vi "Main Page.vi"(8 "error in (no error)":errorcluster, 11 "Node Ptr":T1 format="%.0x") -> (0 "error out":errorcluster)   [LabVIEW 2017, in "NI-SWITCH System Explorer.lvlib"]
uses:
  NI-SWITCH System Explorer.lvlib
  <vilib>/NI Veristand/Custom Device API/Custom Device Item Ref.ctl
  Main Page Controls.ctl
  <vilib>/NI VeriStand/Custom Device API/Custom Device API.lvlib
  Scripting/NI-SWITCH Scripting.lvlib
panel:
  out "Normally Connected Information":cluster{"String":string}={"String"="This topology contains endpoints which are normally connected. See the documentation for more information."}
  in  "Custom Device Name":string
  in  "Topology":string(combo)
  in  "Resource":string
  in  "SHDocVw.IWebBrowser":refnum<k7>(container)
  in  "Description":string
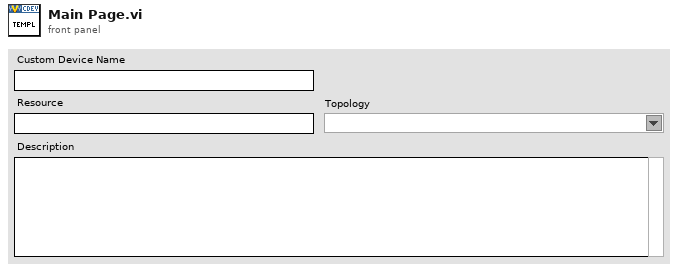
[diagram p1: front panel]
types:
  T1 = typedef "Custom Device API.lvlib/Custom Device Item Ref.ctl" = u64
  T2 = typedef "NI-SWITCH System Explorer.lvlib/Main Page Controls.ctl" = cluster{"Name":refnum<vi>, "Description":refnum<vi>, "Resource":refnum<vi>, "Topology":refnum<vi>, "Normally Connected Information":refnum<vi>}
  T3 = typedef "Custom Device API.lvlib/Custom Device Commands.ctl" = enum16{"Default", "Item renamed", "Shutdown", "Dynamic button pressed"}
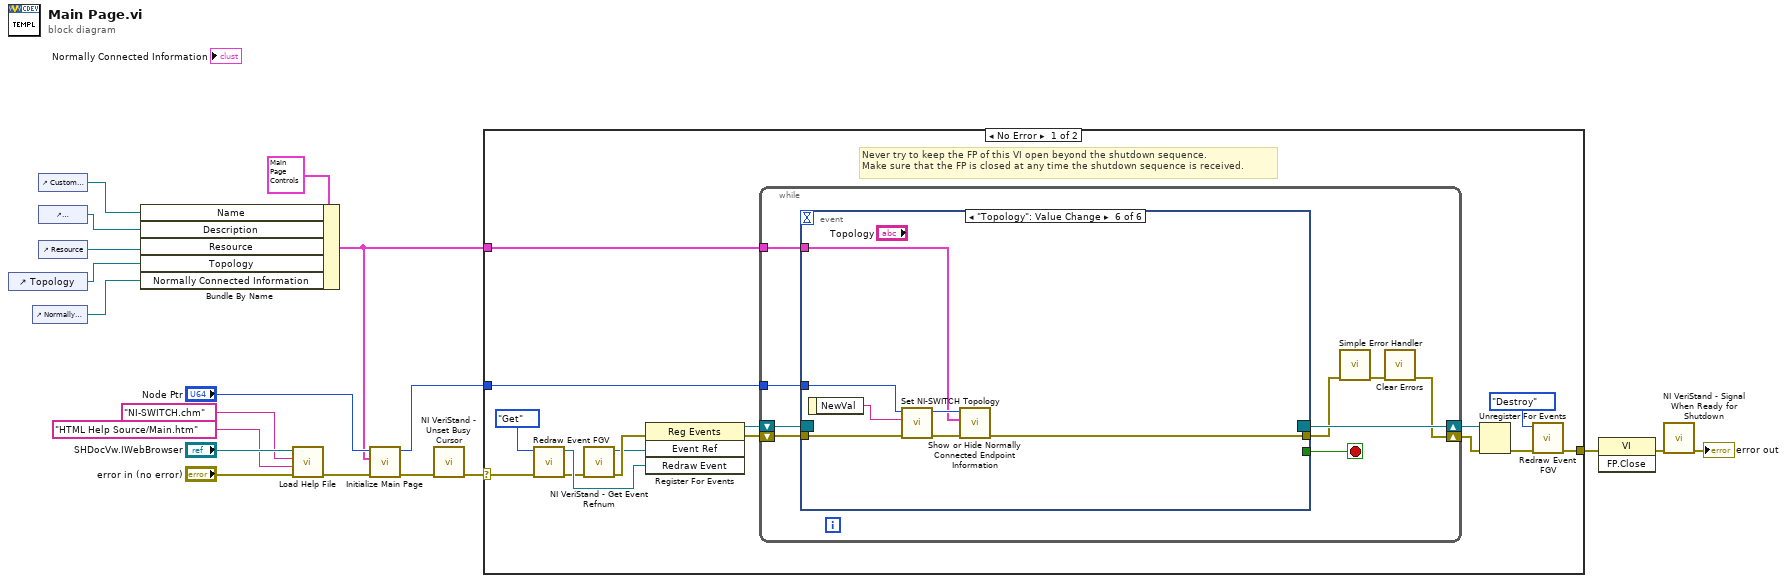
[diagram p0: block diagram]
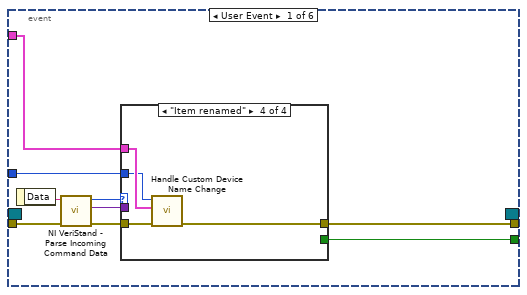
[diagram p2: hidden frame]
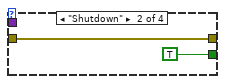
[diagram p4: hidden frame]
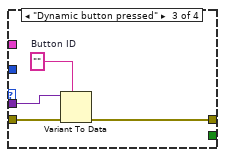
[diagram p5: hidden frame]
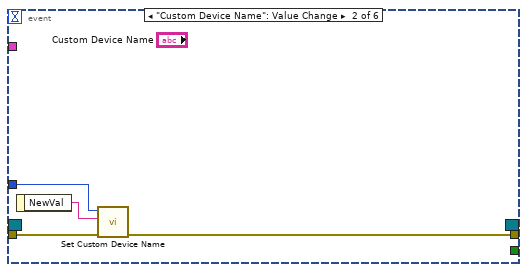
[diagram p6: hidden frame]
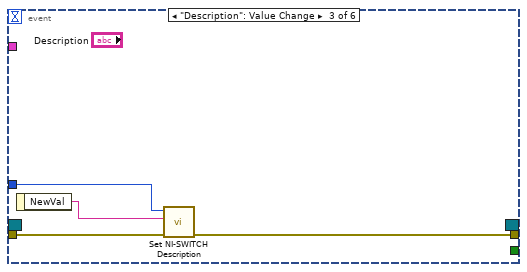
[diagram p7: hidden frame]
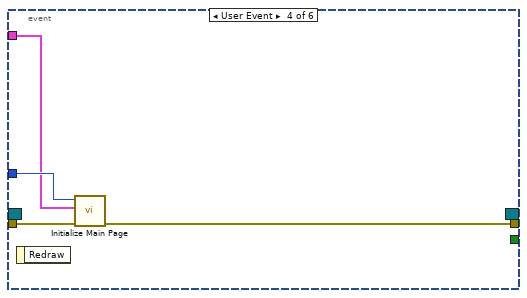
[diagram p8: hidden frame]
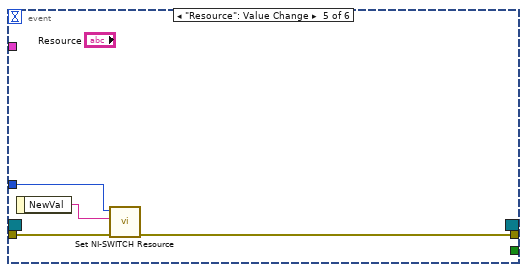
[diagram p9: hidden frame]
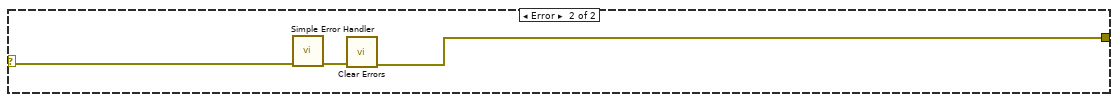
[diagram p10: hidden frame]
diagram:
  n1 = control-ref of="Topology"() -> (w5:refnum<vi>)
  n2 = control-ref of="Normally Connected Information"() -> (w1:refnum<vi>)
  n3 = control-ref of="Custom Device Name"() -> (w2:refnum<vi>)
  n4 = control-ref of="Description"() -> (w8:refnum<vi>)
  n5 = control-ref of="Resource"() -> (w4:refnum<vi>)
  n6 = Bundle By Name(cluster=T2 {"Name"=refnum, "Description"=refnum, "Resource"=refnum, "Topology"=refnum, "Normally Connected Information"=refnum} ("Main Page Controls"), "Name"=w2, "Description"=w8, "Resource"=w4, "Topology"=w5, "Normally Connected Information"=w1) -> (w3:T2)
  n7 = call "Load Help File.vi"("error in (no error)"="error in (no error)", "HTML File to Load"="HTML Help Source/Main.htm" ("HTML File"), "Main CHM File"="NI-SWITCH.chm" ("CD_CHM_FileName"), "Browser"="SHDocVw.IWebBrowser") -> ("error out"=w6:errorcluster)  [unwired: 7 in]
  n8 = call "Initialize Main Page.vi"("error in (no error)"=w6, "Main Page Controls"=w3, "Item Ref in"="Node Ptr") -> ("error out"=w15:errorcluster, "Item Ref out"=w12:T1)  [unwired: 7 in]
  n9 = call <vilib>:"NI VeriStand - Unset Busy Cursor.vi"("error in (no error)"=w15) -> ("error out"=w14:errorcluster)  [unwired: 10 out]
  n10 = case shown="No Error" w14 {
    selector: w14 -> [w22 w89]
    tunnel: [w24 w87] -> w19
    tunnel: w12 -> [w28 _]
    tunnel: w3 -> [w26 _]
    frame No Error {
      # "Never try to keep the FP of this VI open beyond the shutdown sequence.\nMake sure that the FP is closed at any time the shutdown sequence is received."
      n11 = call "Redraw Event FGV.vi"("error in (no error)"=w22, "Action (Get)"=enum16{"Get", "Destroy"}."Get") -> ("error out"=w21:errorcluster, "Redraw Event"=w27:refnum<user-event>)  [unwired: 8 in]
      n12 = call <vilib>:"NI VeriStand - Get Event Refnum.vi"("error in (no error)"=w21) -> ("error out"=w34:errorcluster, "Event Ref"=w31:refnum<user-event>)  [unwired: 9 out]
      n13 = register-events(error in=w34, w31, w27) -> (reference out=w29:refnum<event-registration>, error out=w30:errorcluster)  [unwired: 1 in]
      n14 = while {
        tunnel: w28 -> [w39]
        shift-right: [w36] -> w32
        shift-left: w30 -> [w42]
        shift-right: [w43] -> w33
        shift-left: w29 -> [w41]
        tunnel: w26 -> [w35]
        stop <- w40 stop-if-true
        n15 = event shown="[5] \"Topology\": Value Change" {
          selector: w41 -> [_ _ _ _ _ _]
          dyn-events: [_ _ _ _ _ _] -> w43
          timeout: _ -> [_ _ _ _ _ _]
          tunnel: w42 -> [w52 w67 w70 w73 w79 w86]
          tunnel: [w48 _ _ _ _ _] -> w40
          tunnel: [w47 w66 w69 w72 w76 w82] -> w38
          tunnel: w39 -> [w46 w65 w71 w75 w78 w85]
          tunnel: w35 -> [w44 _ _ w74 _ w80]
          event User Event {
            n16 = event-data() -> ("Data"=w51:string)  [unwired: 1 out]
            n17 = call <vilib>:"NI VeriStand - Parse Incoming Command Data.vi"("error in (no error)"=w52, "Incoming data"=w51) -> ("error out"=w50:errorcluster, "Outgoing data"=w45:variant, "Action"=w49:T3)  [unwired: 7 out]
            n18 = case shown="\"Item renamed\"" w49 {
              tunnel: w50 -> [w53 w54 w59 w63]
              tunnel: [_ TRUE _ _] -> w48
              tunnel: [w53 w54 w56 w62] -> w47
              tunnel: w46 -> [_ _ _ w60]
              tunnel: w45 -> [_ _ w58 _]
              tunnel: w44 -> [_ _ _ w61]
              frame "Default", Default {
              }
              frame "Shutdown" {
              }
              frame "Dynamic button pressed" {
                w57 = ""  # Button ID
                n19 = Variant To Data(error in=w59, type=w57, Variant=w58) -> (error out=w56:errorcluster)  [unwired: 1 out]
              }
              frame "Item renamed" {
                n20 = call "Handle Custom Device Name Change.vi"("error in (no error)"=w63, "Main Page Controls"=w61, "Item Ref in"=w60) -> ("error out"=w62:errorcluster)  [unwired: 7 in, 1 out]
              }
            }
          }
          event "Custom Device Name": Value Change {
            n21 = event-data() -> ("NewVal"=w64:string)  [unwired: 1 out]
            n22 = call "Set Custom Device Name.vi"("error in"=w67, "name"=w64, "ni-switch custom device in"=w65) -> ("error out"=w66:errorcluster)  [unwired: 6 in, 1 out]
          }
          event "Description": Value Change {
            n23 = event-data() -> ("NewVal"=w68:string)  [unwired: 1 out]
            n24 = call "Set NI-SWITCH Description.vi"("error in"=w70, "description"=w68, "ni-switch custom device in"=w71) -> ("error out"=w69:errorcluster)  [unwired: 7 in, 1 out]
          }
          event User Event {
            n25 = event-data() -> ()  [unwired: 2 out]
            n26 = call "Initialize Main Page.vi"("error in (no error)"=w73, "Main Page Controls"=w74, "Item Ref in"=w75) -> ("error out"=w72:errorcluster)  [unwired: 7 in, 1 out]
          }
          event "Resource": Value Change {
            n27 = event-data() -> ("NewVal"=w77:string)  [unwired: 1 out]
            n28 = call "Set NI-SWITCH Resource.vi"("error in"=w79, "resource"=w77, "ni-switch custom device in"=w78) -> ("error out"=w76:errorcluster)  [unwired: 7 in, 1 out]
          }
          event "Topology": Value Change {
            n29 = event-data() -> ("NewVal"=w84:string)  [unwired: 1 out]
            n30 = call "Set NI-SWITCH Topology.vi"("error in"=w86, "topology"=w84, "ni-switch custom device in"=w85) -> ("error out"=w83:errorcluster, "ni-switch custom device out"=w81:T1)  [unwired: 7 in]
            n31 = call "Show or Hide Normally Connected Endpoint Information.vi"("error in (no error)"=w83, "Main Page Controls"=w80, "ni-switch custom device in"=w81) -> ("error out"=w82:errorcluster)  [unwired: 7 in, 1 out]
          }
        }
        n32 = call <vilib>:"Simple Error Handler.vi"("error in (no error)"=w38) -> ("error out"=w37:errorcluster)  [unwired: 1 in, 7 out]
        n33 = call <vilib>:"Clear Errors.vi"("error in (no error)"=w37) -> ("error out"=w36:errorcluster)  [unwired: 1 in, 5 out]
      }
      n34 = Unregister For Events(event registration refnum=w33, error in=w32) -> (error out=w25:errorcluster)
      n35 = call "Redraw Event FGV.vi"("error in (no error)"=w25, "Action (Get)"=enum16{"Get", "Destroy"}."Destroy") -> ("error out"=w24:errorcluster)  [unwired: 8 in, 1 out]
    }
    frame Error {
      n36 = call <vilib>:"Simple Error Handler.vi"("error in (no error)"=w89) -> ("error out"=w88:errorcluster)  [unwired: 1 in, 7 out]
      n37 = call <vilib>:"Clear Errors.vi"("error in (no error)"=w88) -> ("error out"=w87:errorcluster)  [unwired: 1 in, 5 out]
    }
  }
  n38 = invoke class="VI" method="FP.Close"(error in=w19) -> (error out=w18:errorcluster)  [unwired: 2 in, 2 out]
  n39 = call <vilib>:"NI VeriStand - Signal When Ready for Shutdown.vi"("error in (no error)"=w18) -> ("error out"=→"error out":errorcluster)  [unwired: 10 out]
